vi "maintain current instructions.vi"(6 "error in (no error)":errorcluster, 9 "running commands":string[][](array[string])) -> (0 "error out":errorcluster, 3 "running commands out":string[][](array[string]))   [LabVIEW 2011]
uses:
  <vilib>/addons/control/pid/pid.llb/PID (DBL).vi
  VisionData.vi
  <vilib>/addons/control/pid/NI_PID_pid.lvlib
panel:
  in  "visionDrive output range":cluster{"output high":dbl, "output low":dbl}={"output high"=0.3, "output low"=-0.3} {"output low" format="%.2f"; "output high" format="%.2f"}
  in  "visionDrive PID":T1={"proportional gain (Kc)"=-2.5, "integral time (Ti, min)"=0.0, "derivative time (Td, min)"=0.0} {"derivative time (Td, min)" format="%.3f"; "integral time (Ti, min)" format="%.3f"; "proportional gain (Kc)" format="%.3f"}
  in  "y":dbl=100.0
  out "Numeric":dbl
  in  "manualDrivePID":T1={"proportional gain (Kc)"=1.0, "integral time (Ti, min)"=0.01, "derivative time (Td, min)"=0.0} {"derivative time (Td, min)" format="%.3f"; "integral time (Ti, min)" format="%.3f"; "proportional gain (Kc)" format="%.3f"}
  in  "basicDrive PID":T1={"proportional gain (Kc)"=0.03, "integral time (Ti, min)"=0.01, "derivative time (Td, min)"=0.0} {"derivative time (Td, min)" format="%.3f"; "integral time (Ti, min)" format="%.3f"; "proportional gain (Kc)" format="%.3f"}
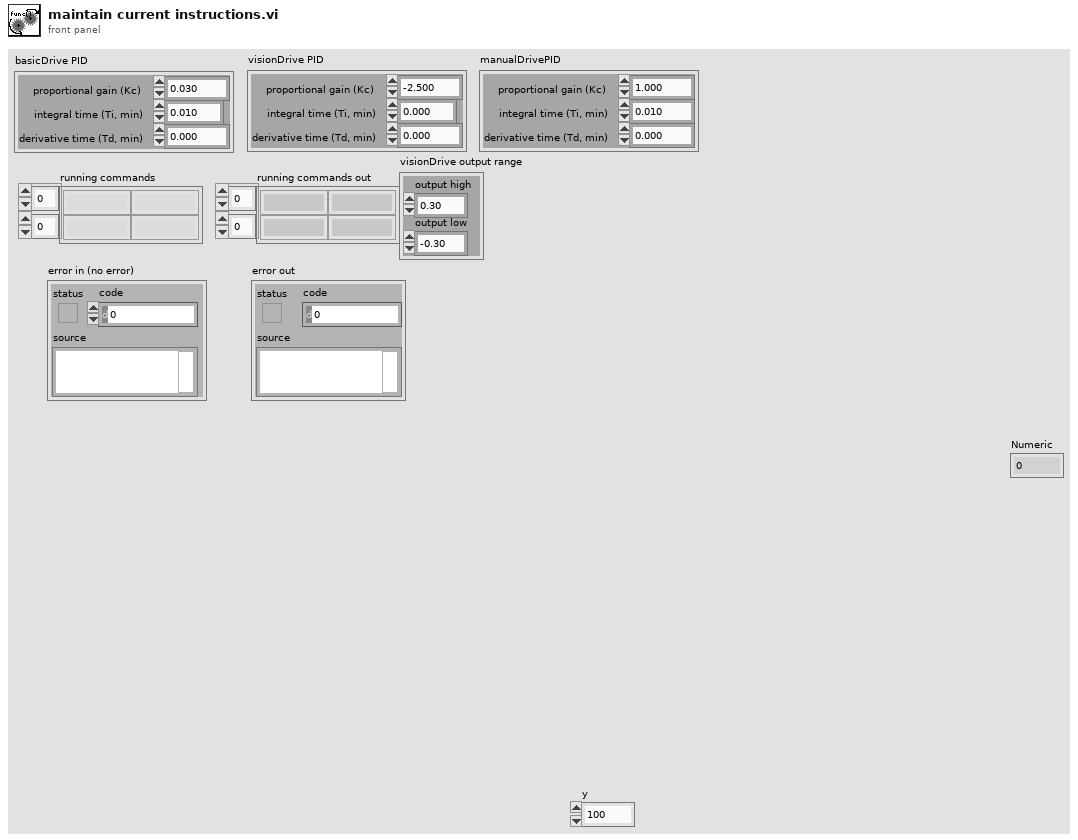
[diagram p1: front panel]
types:
  T1 = cluster{"proportional gain (Kc)":dbl, "integral time (Ti, min)":dbl, "derivative time (Td, min)":dbl}
  T2 = typedef "WPI_EncoderDevRef.ctl" = cluster{"DevStatus":errorcluster, "EncoderIndex":T3, "CounterIndex":T4, "DistancePerCount":dbl, "Decoding Type":T5}
  T3 = typedef "FPGA_EncoderIdx.ctl" = enum8{"Enc 0", "Enc 1", "Enc 2", "Enc 3", "Invalid"}
  T4 = typedef "FPGA_CounterCtrSystemIndex.ctl" = enum8{"Ctr 0", "Ctr 1", "Ctr 2", "Ctr 3", "Ctr 4", "Ctr 5", "Ctr 6", "Ctr 7", "Invalid"}
  T5 = typedef "WPI_EncoderType.ctl" = enum16{"1x", "2x", "4x"}
  T6 = cluster{"Position":cluster{"X":dbl, "Y":dbl}, "Distance (ft)":dbl, "NoTarget":bool, "Right":bool, "Center":bool, "Left":bool, "-1 to 1 CurrentCenter Value":dbl}
  T7 = typedef "WPI_MotorControlDeviceRef.ctl" = cluster{"DeviceStatus":errorcluster, "Type":enum16{"PWM", "CAN"}, "PWM":cluster{"Digital Module":T8, "PWM Channel":T9, "DeadBand":T10}, "CAN":cluster{"Device Number":u8, "Control Mode":T11, "Semaphore":T12, "Max Vout":dbl}, "Invert":bool, "TransformRef":T13, "InvTransformRef":T13}
  T8 = typedef "FPGA_TypedefDigitalModule.ctl" = enum16{"Digital Module 1", "Digital Module 2"}
  T9 = typedef "FPGA_DIOPWMChannel.ctl" = enum8{"PWM 1", "PWM 2", "PWM 3", "PWM 4", "PWM 5", "PWM 6", "PWM 7", "PWM 8", "PWM 9", "PWM 10", "Invalid"}
  T10 = typedef "WPI_PWMDeadband.ctl" = cluster{"Name":string, "maxPositivePwm":i32, "minPositivePwm":i32, "centerPwm":i32, "maxNegativePwm":i32, "minNegativePwm":i32, "angularRange":u16}
  T11 = typedef "WPI_CANJaguar_ControlMode.ctl" = enum8{"Percent VBus", "Current", "Speed", "Position", "Voltage"}
  T12 = typedef "Semaphore RefNum" = refnum<k1>
  T13 = typedef "WPI_PWMTransform_ConPane.ctl" = refnum<vi>
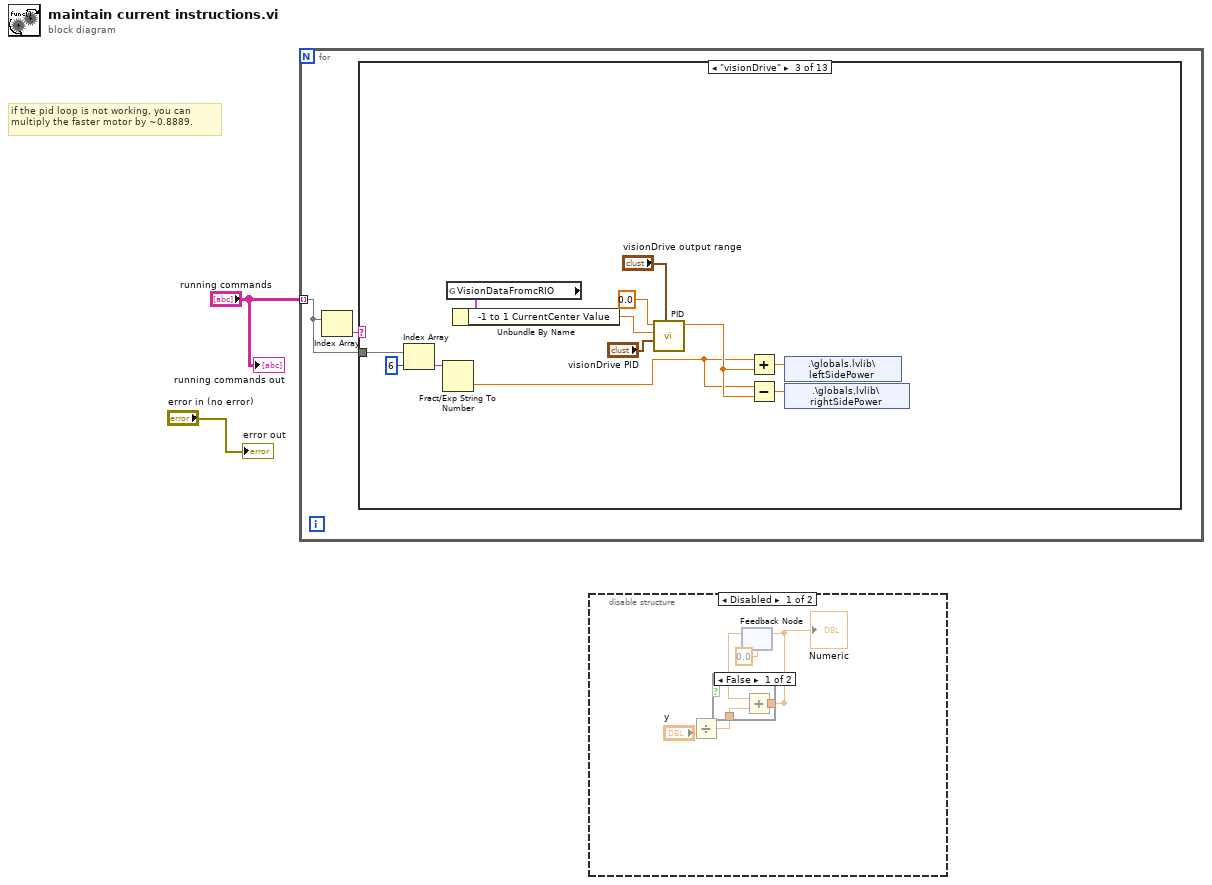
[diagram p0: block diagram]
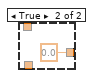
[diagram p2: hidden frame]
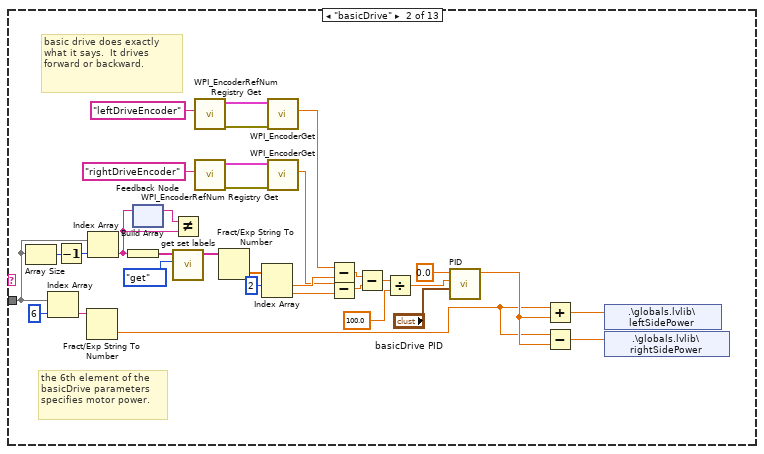
[diagram p5: hidden frame]
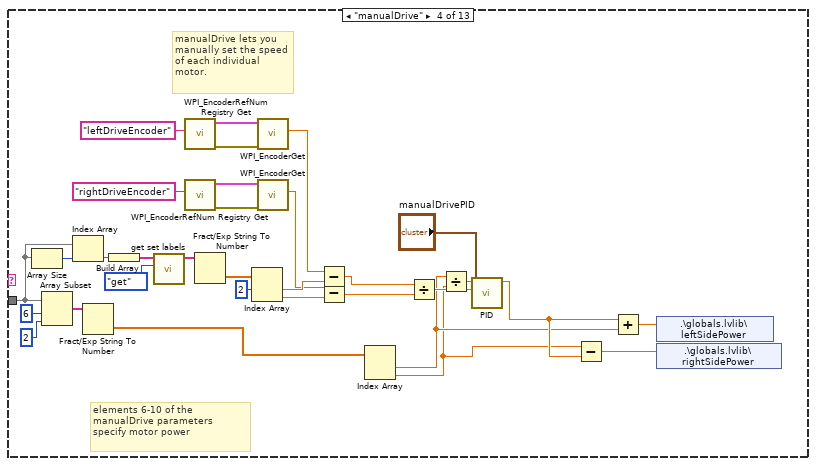
[diagram p6: hidden frame]
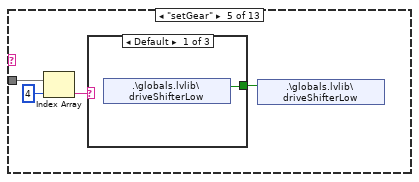
[diagram p7: hidden frame]
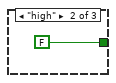
[diagram p8: hidden frame]
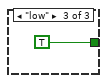
[diagram p9: hidden frame]
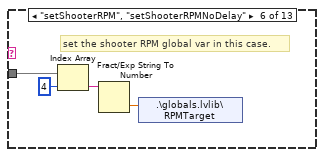
[diagram p10: hidden frame]
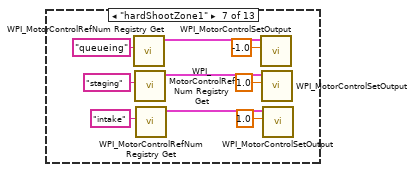
[diagram p11: hidden frame]
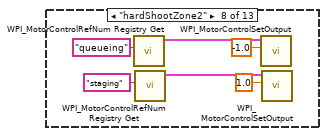
[diagram p12: hidden frame]
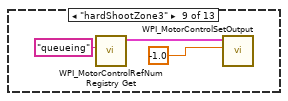
[diagram p13: hidden frame]
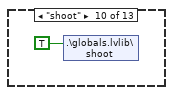
[diagram p14: hidden frame]
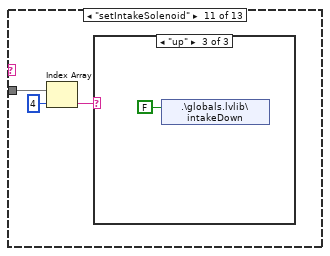
[diagram p15: hidden frame]
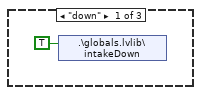
[diagram p16: hidden frame]
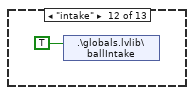
[diagram p18: hidden frame]
diagram:
  # "if the pid loop is not working, you can multiply the faster motor by ~0.8889."
  n1 = for {
    tunnel: "running commands" -> [w3] mode=indexing
    n2 = Index Array(array=w3) -> (element=w4:string)  [unwired: 1 in]
    n3 = case shown="\"visionDrive\"" w4 {
      tunnel: w3 -> [_ w19 w41 w73 w85 w92 _ _ _ _ w113 _ _]
      frame Default {
      }
      frame "basicDrive" {
        # "basic drive does exactly what it says.  It drives forward or backward."
        # "the 6th element of the basicDrive parameters specifies motor power."
        n4 = Array Size(array=w19) -> (size(s)=w12:i32)
        n5 = Index Array(array=w19, index=6) -> (element=w36:string)
        n6 = Decrement(x=w12) -> (x-1=w11:i32)
        n7 = Fract/Exp String To Number(string=w36) -> (number=w7:dbl)  [unwired: 3 in, 1 out]
        n8 = Index Array(array=w19, index=w11) -> (element=w13:string)
        n9 = Build Array(w13) -> (w34:string[])
        n10 = feedback #1() -> (w14:string)  [unwired: 1 in]
        n11 = feedback-in #1(w13) -> ()
        n12 = Not Equal?(x=w14, y=w13) -> ()  [unwired: 1 out]
        n13 = call "get set labels.vi"("option in"=enum16{"get", "set", "remove", "set end"}."get", "label in"=w34) -> ("label out"=w26:string[])  [unwired: 9 in]
        n14 = call <vilib>:"WPI_EncoderRefNum Registry Get.vi"("refnum name"="leftDriveEncoder") -> ("error out"=w32:errorcluster, "EncoderDevRef"=w33:T2)  [unwired: 9 in]
        n15 = call <vilib>:"WPI_EncoderRefNum Registry Get.vi"("refnum name"="rightDriveEncoder") -> ("error out"=w29:errorcluster, "EncoderDevRef"=w28:T2)  [unwired: 9 in]
        n16 = Fract/Exp String To Number(string=w26) -> (number=w25:dbl[])  [unwired: 3 in, 1 out]
        n17 = Index Array(array=w25, index #1=2 ("index")) -> (element #1=w23:dbl, element #2=w21:dbl)  [unwired: 1 in]
        n18 = call <vilib>:"WPI_EncoderGet.vi"("error in (no error)"=w32, "EncoderDevRef"=w33) -> ("Distance"=w24:dbl)  [unwired: 4 in, 5 out]
        n19 = call <vilib>:"WPI_EncoderGet.vi"("error in (no error)"=w29, "EncoderDevRef"=w28) -> ("Distance"=w22:dbl)  [unwired: 4 in, 5 out]
        n20 = Subtract(x=w24, y=w23) -> (x-y=w8:dbl)
        n21 = Subtract(x=w22, y=w21) -> (x-y=w9:dbl)
        n22 = Subtract(x=w8, y=w9) -> (x-y=w18:dbl)
        n23 = Divide(x=w18, y=100.0) -> (x/y=w16:dbl)
        n24 = call-poly <vilib>:"PID.vi"("PID gains"="basicDrive PID", "process variable"=w16, "setpoint"=0.0) -> ("output"=w10:dbl)  [unwired: 7 in, 1 out]
        n25 = Add(x=w7, y=w10) -> (x+y=w6:dbl)
        n26 = Subtract(x=w7, y=w10) -> (x-y=w5:dbl)
        n27 = shared-variable ".\\globals.lvlib\\leftSidePower"(w6) -> ()  [unwired: 1 in, 1 out]
        n28 = shared-variable ".\\globals.lvlib\\rightSidePower"(w5) -> ()  [unwired: 1 in, 1 out]
      }
      frame "visionDrive" {
        n29 = Index Array(array=w41, index=6) -> (element=w48:string)
        n30 = Fract/Exp String To Number(string=w48) -> (number=w44:dbl)  [unwired: 3 in, 1 out]
        n31 = global read "VisionData.vi" "VisionDataFromcRIO"() -> (w40:T6)
        n32 = Unbundle By Name(w40) -> ("-1 to 1 CurrentCenter Value"=w39:dbl)
        n33 = call-poly <vilib>:"PID.vi"("output range"="visionDrive output range", "PID gains"="visionDrive PID", "process variable"=w39, "setpoint"=0.0) -> ("output"=w45:dbl)  [unwired: 6 in, 1 out]
        n34 = Add(x=w44, y=w45) -> (x+y=w43:dbl)
        n35 = Subtract(x=w44, y=w45) -> (x-y=w42:dbl)
        n36 = shared-variable ".\\globals.lvlib\\leftSidePower"(w43) -> ()  [unwired: 1 in, 1 out]
        n37 = shared-variable ".\\globals.lvlib\\rightSidePower"(w42) -> ()  [unwired: 1 in, 1 out]
      }
      frame "manualDrive" {
        # "manualDrive lets you manually set the speed of each individual motor."
        # "elements 6-10 of the manualDrive parameters specify motor power"
        n38 = Array Size(array=w73) -> (size(s)=w75:i32)
        n39 = Array Subset(array=w73, index=6, length=2) -> (w79:string[])
        n40 = Index Array(array=w73, index=w75) -> (element=w74:string)
        n41 = Fract/Exp String To Number(string=w79) -> (number=w78:dbl[])  [unwired: 3 in, 1 out]
        n42 = Build Array(w74) -> (w76:string[])
        n43 = call "get set labels.vi"("option in"=enum16{"get", "set", "remove", "set end"}."get", "label in"=w76) -> ("label out"=w65:string[])  [unwired: 9 in]
        n44 = call <vilib>:"WPI_EncoderRefNum Registry Get.vi"("refnum name"="leftDriveEncoder") -> ("error out"=w71:errorcluster, "EncoderDevRef"=w72:T2)  [unwired: 9 in]
        n45 = call <vilib>:"WPI_EncoderRefNum Registry Get.vi"("refnum name"="rightDriveEncoder") -> ("error out"=w68:errorcluster, "EncoderDevRef"=w67:T2)  [unwired: 9 in]
        n46 = Fract/Exp String To Number(string=w65) -> (number=w64:dbl[])  [unwired: 3 in, 1 out]
        n47 = Index Array(array=w64, index #1=2 ("index")) -> (element #1=w62:dbl, element #2=w60:dbl)  [unwired: 1 in]
        n48 = call <vilib>:"WPI_EncoderGet.vi"("error in (no error)"=w71, "EncoderDevRef"=w72) -> ("Distance"=w63:dbl)  [unwired: 4 in, 5 out]
        n49 = call <vilib>:"WPI_EncoderGet.vi"("error in (no error)"=w68, "EncoderDevRef"=w67) -> ("Distance"=w61:dbl)  [unwired: 4 in, 5 out]
        n50 = Subtract(x=w63, y=w62) -> (x-y=w57:dbl)
        n51 = Subtract(x=w61, y=w60) -> (x-y=w56:dbl)
        n52 = Index Array(array=w78) -> (element #1=w52:dbl, element #2=w51:dbl)  [unwired: 2 in]
        n53 = Divide(x=w57, y=w56) -> (x/y=w59:dbl)
        n54 = Divide(x=w52, y=w51) -> (x/y=w58:dbl)
        n55 = call-poly <vilib>:"PID.vi"("PID gains"="manualDrivePID", "process variable"=w59, "setpoint"=w58) -> ("output"=w53:dbl)  [unwired: 7 in, 1 out]
        n56 = Subtract(x=w51, y=w53) -> (x-y=w50:dbl)
        n57 = Add(x=w53, y=w52) -> (x+y=w54:dbl)
        n58 = shared-variable ".\\globals.lvlib\\leftSidePower"(w54) -> ()  [unwired: 1 in, 1 out]
        n59 = shared-variable ".\\globals.lvlib\\rightSidePower"(w50) -> ()  [unwired: 1 in, 1 out]
      }
      frame "setGear" {
        n60 = Index Array(array=w85, index=4) -> (element=w84:string)
        n61 = case shown="Default" w84 {
          tunnel: [w86 FALSE ("driveShifterLow") TRUE ("driveShifterLow")] -> w83
          frame Default {
            n62 = shared-variable ".\\globals.lvlib\\driveShifterLow"() -> (w86:bool)  [unwired: 1 in, 1 out]
          }
          frame "high" {
          }
          frame "low" {
          }
        }
        n63 = shared-variable ".\\globals.lvlib\\driveShifterLow"(w83) -> ()  [unwired: 1 in, 1 out]
      }
      frame "setShooterRPM", "setShooterRPMNoDelay" {
        # "set the shooter RPM global var in this case."
        n64 = Index Array(array=w92, index=4) -> (element=w90:string)
        n65 = Fract/Exp String To Number(string=w90) -> (number=w89:dbl)  [unwired: 3 in, 1 out]
        n66 = shared-variable ".\\globals.lvlib\\RPMTarget"(w89) -> ()  [unwired: 1 in, 1 out]
      }
      frame "hardShootZone1" {
        n67 = call <vilib>:"WPI_MotorControlRefNum Registry Get.vi"("refnum name"="queueing") -> ("MotorControlDevRef"=w97:T7)  [unwired: 9 in, 1 out]
        n68 = call <vilib>:"WPI_MotorControlRefNum Registry Get.vi"("refnum name"="staging") -> ("MotorControlDevRef"=w98:T7)  [unwired: 9 in, 1 out]
        n69 = call <vilib>:"WPI_MotorControlRefNum Registry Get.vi"("refnum name"="intake") -> ("MotorControlDevRef"=w99:T7)  [unwired: 9 in, 1 out]
        n70 = call <vilib>:"WPI_MotorControlSetOutput.vi"("Output"=-1.0, "MotorControlDevRef"=w97) -> ()  [unwired: 8 in, 2 out]
        n71 = call <vilib>:"WPI_MotorControlSetOutput.vi"("Output"=1.0, "MotorControlDevRef"=w98) -> ()  [unwired: 8 in, 2 out]
        n72 = call <vilib>:"WPI_MotorControlSetOutput.vi"("Output"=1.0, "MotorControlDevRef"=w99) -> ()  [unwired: 8 in, 2 out]
      }
      frame "hardShootZone2" {
        n73 = call <vilib>:"WPI_MotorControlRefNum Registry Get.vi"("refnum name"="queueing") -> ("MotorControlDevRef"=w105:T7)  [unwired: 9 in, 1 out]
        n74 = call <vilib>:"WPI_MotorControlRefNum Registry Get.vi"("refnum name"="staging") -> ("MotorControlDevRef"=w106:T7)  [unwired: 9 in, 1 out]
        n75 = call <vilib>:"WPI_MotorControlSetOutput.vi"("Output"=-1.0, "MotorControlDevRef"=w105) -> ()  [unwired: 8 in, 2 out]
        n76 = call <vilib>:"WPI_MotorControlSetOutput.vi"("Output"=1.0, "MotorControlDevRef"=w106) -> ()  [unwired: 8 in, 2 out]
      }
      frame "hardShootZone3" {
        n77 = call <vilib>:"WPI_MotorControlRefNum Registry Get.vi"("refnum name"="queueing") -> ("MotorControlDevRef"=w110:T7)  [unwired: 9 in, 1 out]
        n78 = call <vilib>:"WPI_MotorControlSetOutput.vi"("Output"=-1.0, "MotorControlDevRef"=w110) -> ()  [unwired: 8 in, 2 out]
      }
      frame "shoot" {
        n79 = shared-variable ".\\globals.lvlib\\shoot"(TRUE ("shoot")) -> ()  [unwired: 1 in, 1 out]
      }
      frame "setIntakeSolenoid" {
        n80 = Index Array(array=w113, index=4) -> (element=w112:string)
        n81 = case shown="\"up\"" w112 {
          frame "down" {
            n82 = shared-variable ".\\globals.lvlib\\intakeDown"(TRUE ("intakeDown")) -> ()  [unwired: 1 in, 1 out]
          }
          frame Default {
          }
          frame "up" {
            n83 = shared-variable ".\\globals.lvlib\\intakeDown"(FALSE ("intakeDown")) -> ()  [unwired: 1 in, 1 out]
          }
        }
      }
      frame "intake" {
        n84 = shared-variable ".\\globals.lvlib\\ballIntake"(TRUE ("ballIntake")) -> ()  [unwired: 1 in, 1 out]
      }
      frame "testFunct" {
      }
    }
  }
  n85 = disable-structure shown="Disabled" {
    frame Disabled {
      n86 = Divide(y="y") -> (x/y=w120:dbl)  [unwired: 1 in]
      n87 = feedback #2(0.0) -> (w119:dbl)
      n88 = case shown="False" {
        selector: _ -> [_ _]
        tunnel: w120 -> [w125 _]
        tunnel: w119 -> [w124 _]
        tunnel: [w123 0.0] -> w118
        frame False {
          n89 = Add(x=w124, y=w125) -> (x+y=w123:dbl)
        }
        frame True {
        }
      }
      "Numeric" <- w118
      n90 = feedback-in #2(w118) -> ()
    }
    frame Enabled {
    }
  }
  "running commands out" <- "running commands"
  "error out" <- "error in (no error)"
